vi "Load parameters.vi"(8 "error in (no error)":errorcluster, 11 "Input Cluster":T1) -> (0 "error out":errorcluster)   [LabVIEW 2017]
uses:
  Controls/Testscreen_Input cluster.ctl
  <vilib>/addons/database/Connection.llb/Conn ObjectReference.ctl
  <vilib>/addons/database/NI_Database_API.lvlib
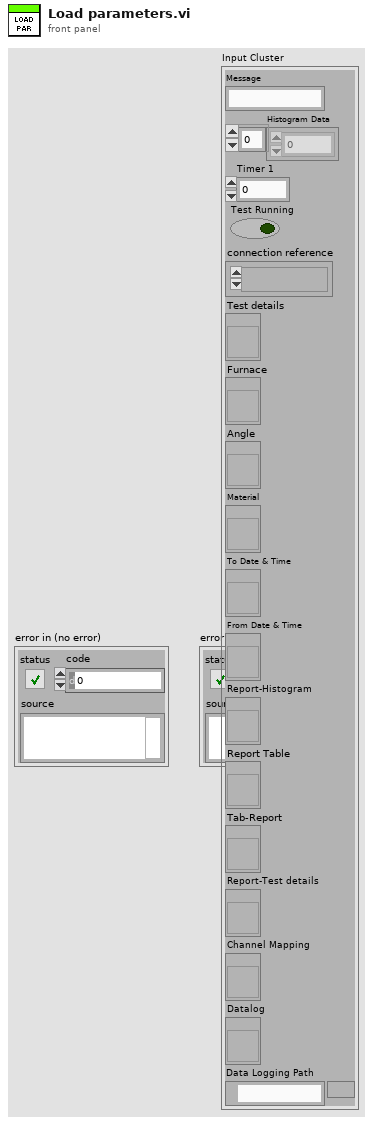
[diagram p1: front panel]
types:
  T1 = typedef "Testscreen_Input cluster.ctl" = cluster{"Message":string, "Histogram Data":i32[], "Timer 1":u32, "Test Running":bool, "connection reference":T2, "Test details":refnum<vi>, "Furnace":refnum<vi>, "Angle":refnum<vi>, "Material":refnum<vi>, "To Date & Time":refnum<vi>, "From Date & Time":refnum<vi>, "Report-Histogram":refnum<vi>, "Report Table":refnum<vi>, "Tab-Report":refnum<vi>, "Report-Test details":refnum<vi>, "Channel Mapping":refnum<vi>, "Datalog":refnum<vi>, "Data Logging Path":path}
  T2 = typedef "NI_Database_API.lvlib/Conn ObjectReference.ctl" = refnum<k1>
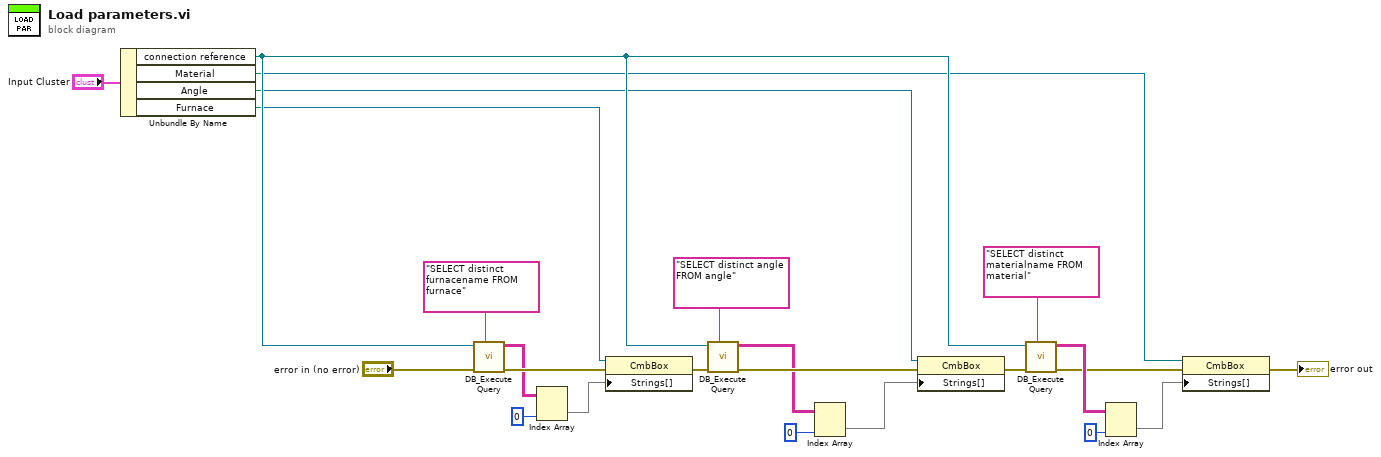
[diagram p0: block diagram]
diagram:
  n1 = Unbundle By Name("Input Cluster") -> ("connection reference"=w4:T2, "Material"=w3:refnum<vi>, "Angle"=w2:refnum<vi>, "Furnace"=w1:refnum<vi>)
  n2 = call "DB_Execute Query.vi"("Query"="SELECT distinct furnacename FROM furnace", "error in (no error)"="error in (no error)", "connection reference"=w4) -> ("error out"=w10:errorcluster, "data"=w7:string[][])  [unwired: 7 in]
  n3 = Index Array(array=w7, index (col)=0 ("disabled index (col)")) -> (element=w9:string[])  [unwired: 1 in]
  n4 = property on="Property Node" class="CmbBox"(reference=w1, error in=w10, "Strings[]"=w9) -> (error out=w13:errorcluster)  [unwired: 1 out]
  n5 = call "DB_Execute Query.vi"("Query"="SELECT distinct angle FROM angle", "error in (no error)"=w13, "connection reference"=w4) -> ("error out"=w16:errorcluster, "data"=w12:string[][])  [unwired: 7 in]
  n6 = Index Array(array=w12, index (col)=0 ("disabled index (col)")) -> (element=w15:string[])  [unwired: 1 in]
  n7 = property on="Property Node" class="CmbBox"(reference=w2, error in=w16, "Strings[]"=w15) -> (error out=w22:errorcluster)  [unwired: 1 out]
  n8 = call "DB_Execute Query.vi"("Query"="SELECT distinct materialname FROM material", "error in (no error)"=w22, "connection reference"=w4) -> ("error out"=w17:errorcluster, "data"=w20:string[][])  [unwired: 7 in]
  n9 = Index Array(array=w20, index (col)=0 ("disabled index (col)")) -> (element=w18:string[])  [unwired: 1 in]
  n10 = property on="Property Node" class="CmbBox"(reference=w3, error in=w17, "Strings[]"=w18) -> (error out=→"error out":errorcluster)  [unwired: 1 out]
